vi "Supercap voltage convertor.vi"(0 "Medición III":string, 1 "Medición 0":string, 2 "Medición II":string, 3 "Medición I":string, 4 "Medición IV":string) -> (5 "Supercap Read II":u32, 6 "Supercap Read IV":u32, 7 "Supercap Read III":u32, 8 "Supercap Read I":u32, 9 "Supercap Read 0":u32)   [LabVIEW 2023]
uses:
  <vilib>/regexp/Match Regular Expression.xnode
panel:
  out "True/False":bool
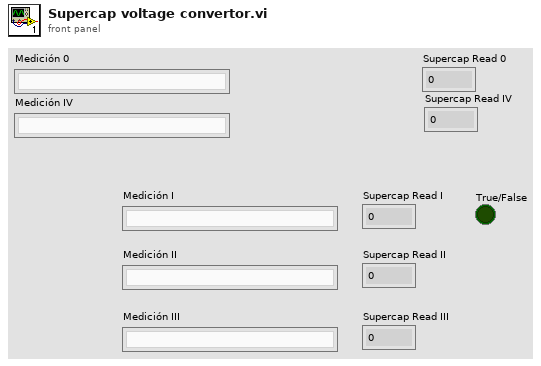
[diagram p1: front panel]
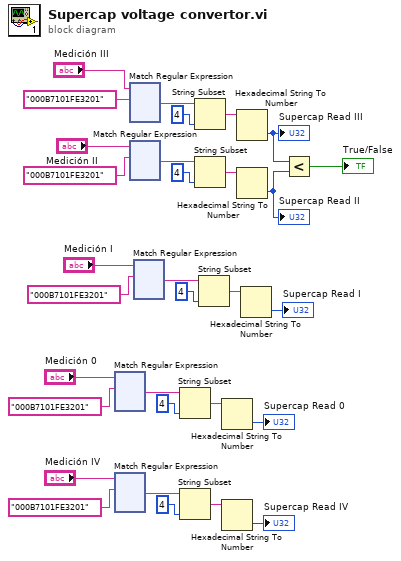
[diagram p0: block diagram]
diagram:
  n1 = xnode "Match Regular Expression"("input string"="Medición 0", "regular expression"="000B7101FE3201") -> ("after match"=w10:string)  [unwired: 4 in, 4 out]
  n2 = xnode "Match Regular Expression"("input string"="Medición IV", "regular expression"="000B7101FE3201") -> ("after match"=w4:string)  [unwired: 4 in, 4 out]
  n3 = xnode "Match Regular Expression"("input string"="Medición III", "regular expression"="000B7101FE3201") -> ("after match"=w17:string)  [unwired: 4 in, 4 out]
  n4 = xnode "Match Regular Expression"("input string"="Medición II", "regular expression"="000B7101FE3201") -> ("after match"=w24:string)  [unwired: 4 in, 4 out]
  n5 = xnode "Match Regular Expression"("input string"="Medición I", "regular expression"="000B7101FE3201") -> ("after match"=w29:string)  [unwired: 4 in, 4 out]
  n6 = String Subset(string=w10, length (rest)=4 ("length (rest)")) -> (substring=w8:string)  [unwired: 1 in]
  n7 = String Subset(string=w4, length (rest)=4 ("length (rest)")) -> (substring=w2:string)  [unwired: 1 in]
  n8 = String Subset(string=w17, length (rest)=4 ("length (rest)")) -> (substring=w15:string)  [unwired: 1 in]
  n9 = String Subset(string=w24, length (rest)=4 ("length (rest)")) -> (substring=w22:string)  [unwired: 1 in]
  n10 = String Subset(string=w29, length (rest)=4 ("length (rest)")) -> (substring=w27:string)  [unwired: 1 in]
  n11 = Hexadecimal String To Number(string=w8) -> (number=→"Supercap Read 0":u32)  [unwired: 2 in, 1 out]
  n12 = Hexadecimal String To Number(string=w2) -> (number=→"Supercap Read IV":u32)  [unwired: 2 in, 1 out]
  n13 = Hexadecimal String To Number(string=w15) -> (number=w14:u32)  [unwired: 2 in, 1 out]
  "Supercap Read III" <- w14
  n14 = Hexadecimal String To Number(string=w22) -> (number=w13:u32)  [unwired: 2 in, 1 out]
  "Supercap Read II" <- w13
  n15 = Hexadecimal String To Number(string=w27) -> (number=→"Supercap Read I":u32)  [unwired: 2 in, 1 out]
  n16 = Less?(x=w14, y=w13) -> (x < y?=→"True/False":bool)
